vi "Main.vi"() -> ()   [LabVIEW 2018]
uses:
  Data Def/Main State.ctl
  Data Def/Tips.ctl
  Data Def/Frequency Setting.ctl
  Data Def/Subpanel State.ctl
  Data Def/Channel Count.ctl
  Data Def/Signal Type Setting.ctl
  Function/Data Def/Voice Control Reference.ctl
  Data Def/Loop Control Command.ctl
  Data Def/Main Loop Command.ctl
  Data Def/Parameter.ctl
  <vilib>/Utility/miscctls.llb/LVPositionTypeDef.ctl
panel:
  in  "Setting Parameter":bool
  in  "Get Data":bool
  in  "Menue":bool
  in  "Score":dbl
  out "Voice Chatt":dbl(graph)
  out "Voice":string
  out "Voice State":bool
  in  "Stop":bool
  in  "Tab Control 2":enum32{"Page 1"}(tab)
  out "Tips":T1
  in  "Help":bool
  out "Main Tab":T2
  in  "Save":bool
  in  "Previous Page":bool
  out "SubTab":T3
  in  "Signal Type":bool
  in  "Channel":bool
  in  "Frequency":bool
  in  "Frequency Setting":T4 caption="頻率"
  in  "Channel Count":T5 caption="通道數"
  in  "Signal Type Setting":T6 caption="波形"
  in  "Switch":bool
  out "Spectrum":cluster{"f0":dbl, "df":dbl, "magnitude":dbl[]}[](graph)
  out "Wave":waveform(dbl)[](graph)
  # "微軟語音辨識軟體動後，請對軟體說出每個\n按鈕的名稱或由左方按鍵手動操作。"
  # "目錄"
  # "請確定微軟語音辨識軟體有正確開啟並運作。"
  # "請選擇以下功能"
  # "設定參數"
  # "擷取數據"
  # "擷取數據"
  # "幫助"
  # "停止"
  # "開/關"
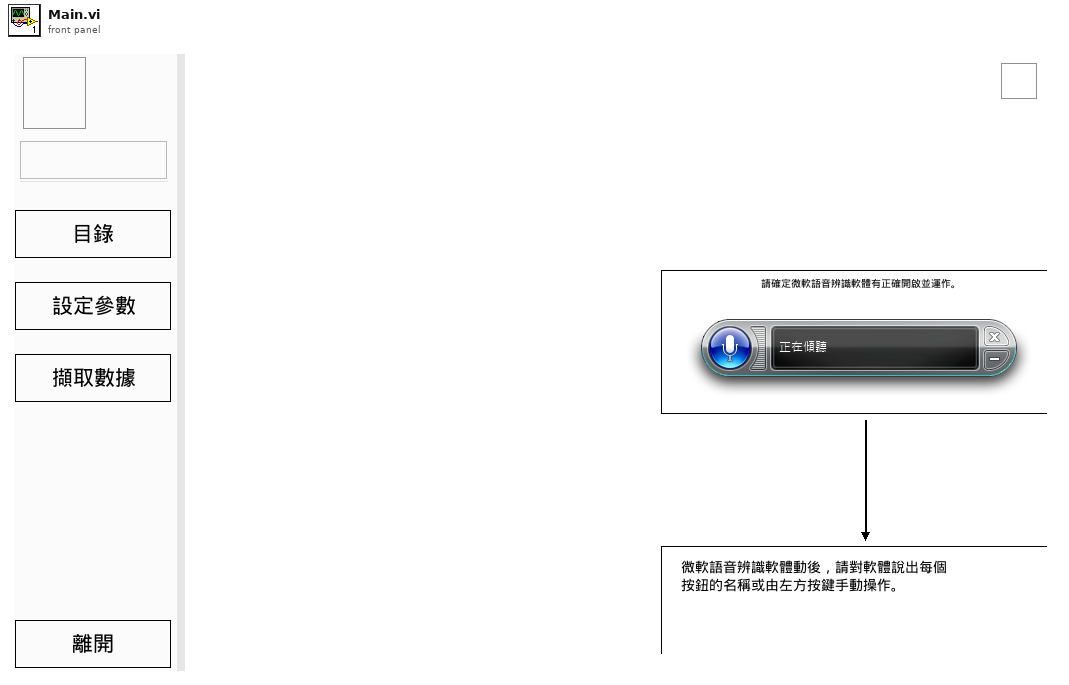
[diagram p1: front panel]
types:
  T1 = typedef "Tips.ctl" = string
  T2 = typedef "Main State.ctl" = enum32{"Initialize", "Start", "Set Parameter", "Get Data"}
  T3 = typedef "Subpanel State.ctl" = enum32{"Main", "Frequency", "Count of Channel", "Signal Type"}
  T4 = typedef "Frequency Setting.ctl" = enum32{"10 Hz", "50 Hz", "100 Hz"}
  T5 = typedef "Channel Count.ctl" = enum32{"1", "2", "3", "4"}
  T6 = typedef "Signal Type Setting.ctl" = enum32{"Sine", "Sqaure", "Triangle"}
  T7 = typedef "Main Loop Command.ctl" = enum16{"Initialize", "Menue", "Setting Parameter", "Get Data", "Help", "Frequency", "Channel", "Signal Type", "Previous Page", "Save", "Exit"}
  T8 = typedef "Loop Control Command.ctl" = enum16{"Initialize", "Enqueue", "Insert", "Flush", "Release"}
  T9 = typedef "Voice Control Reference.ctl" = cluster{"String in":refnum<vi>, "Score in":refnum<vi>}
  T10 = typedef "Callback Event Reference.ctl" = cluster{"new reference":refnum<k24>, "Event Callback":refnum<k27>}
  T11 = enum32{"Main", "Frequency", "Count of Channel", "Signal Type"}
  T12 = typedef "Parameter.ctl" = cluster{"Channel Count":T5, "Frequency Setting":T4, "Signal Type Setting":T6}
  T13 = enum16{"Save File", "Read File", "Put Frequency", "Put Signal Type", "Put Channel", "Put All", "Get All"}
  T14 = typedef "LVPositionTypeDef.ctl" = cluster{"Left":i32, "Top":i32}
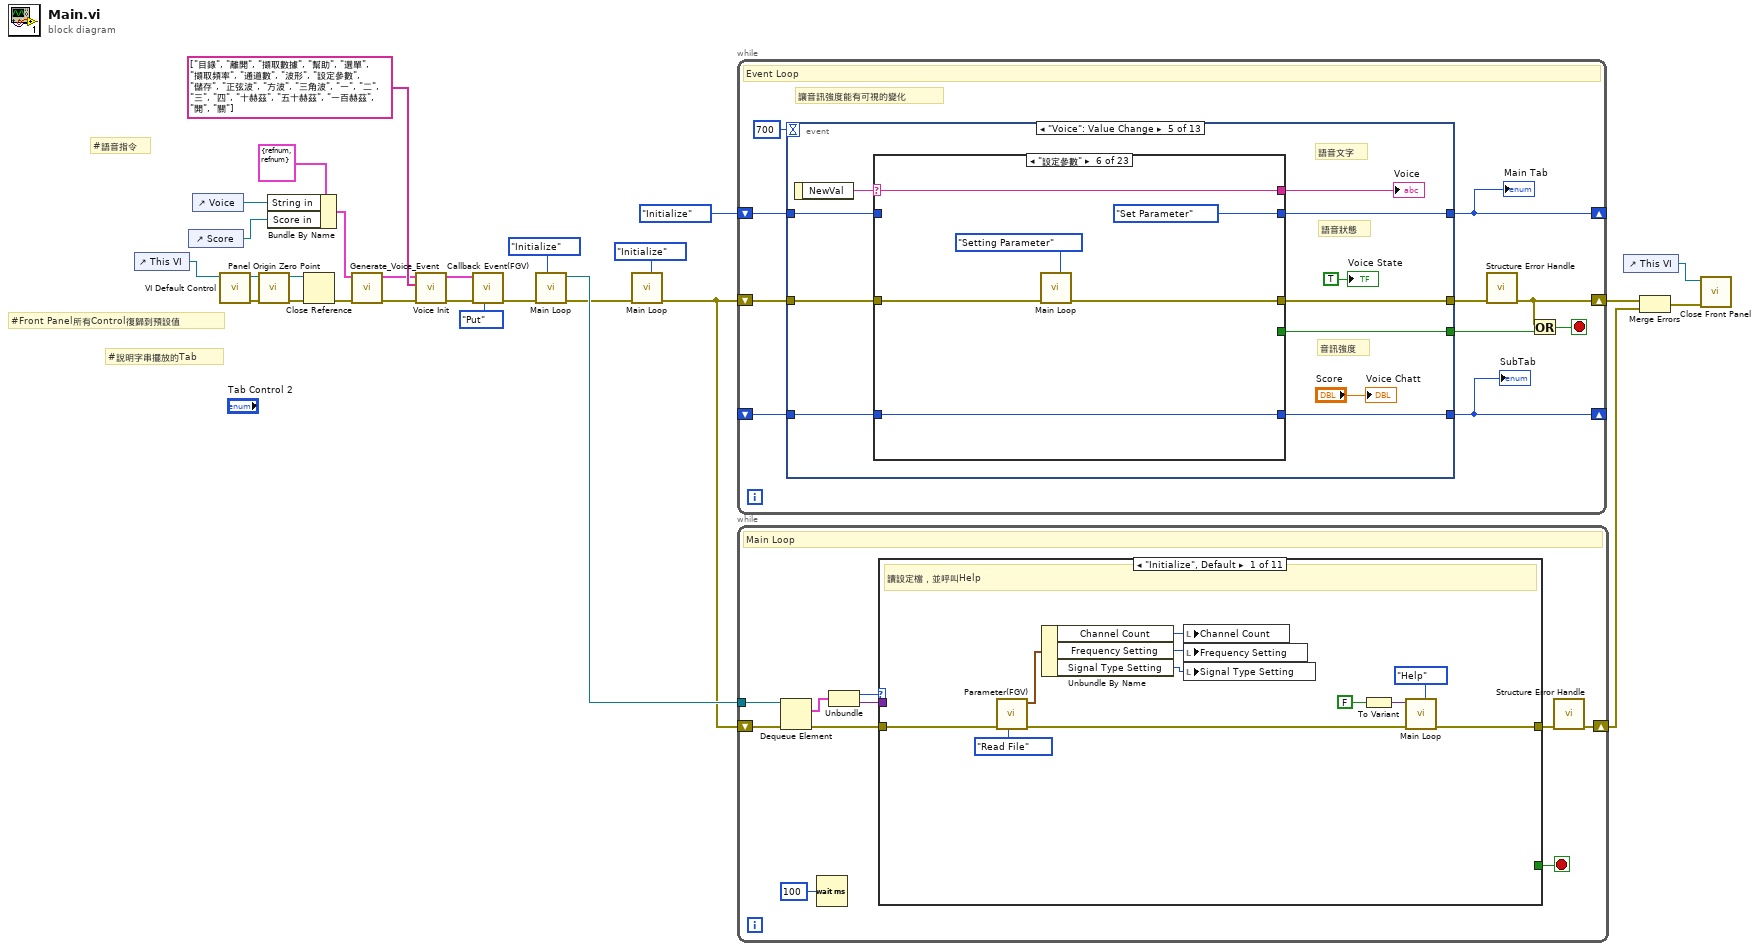
[diagram p0: block diagram]
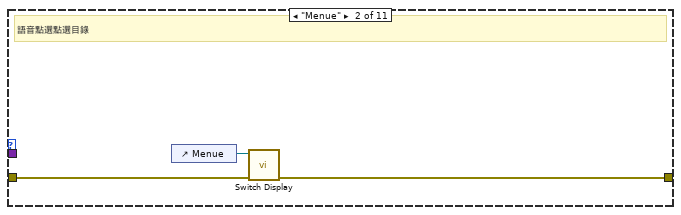
[diagram p2: hidden frame]
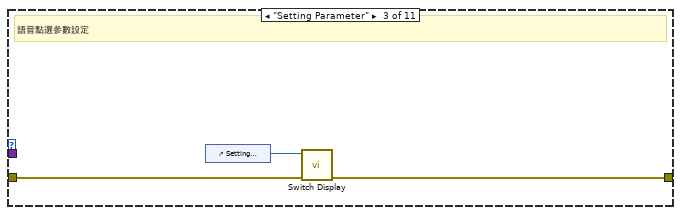
[diagram p3: hidden frame]
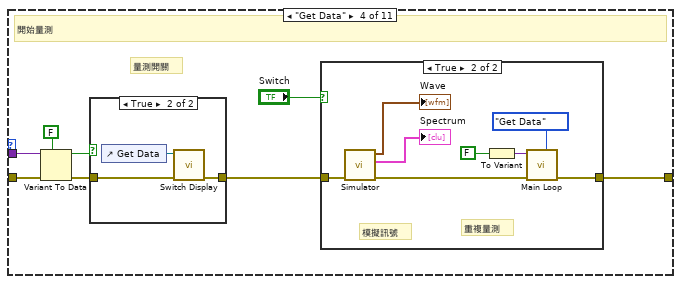
[diagram p4: hidden frame]
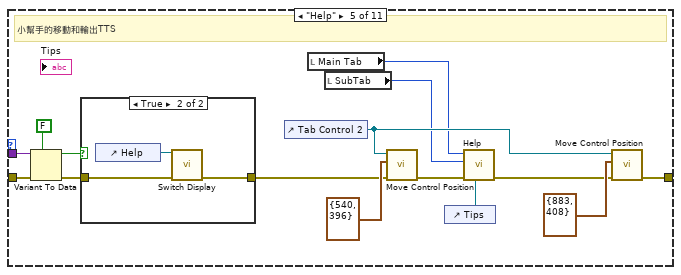
[diagram p7: hidden frame]
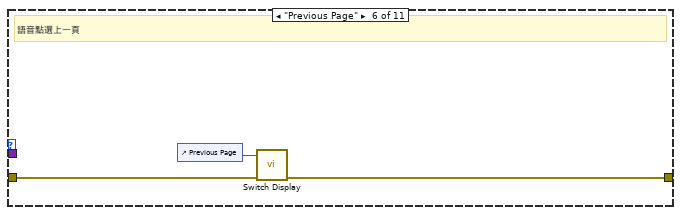
[diagram p9: hidden frame]
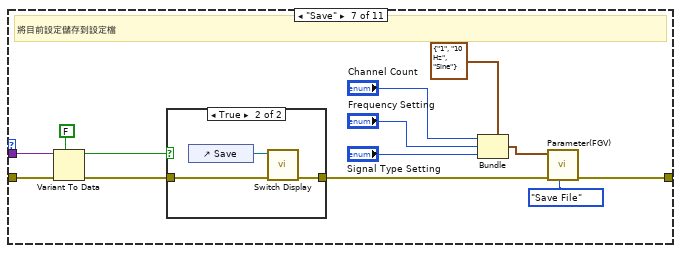
[diagram p10: hidden frame]
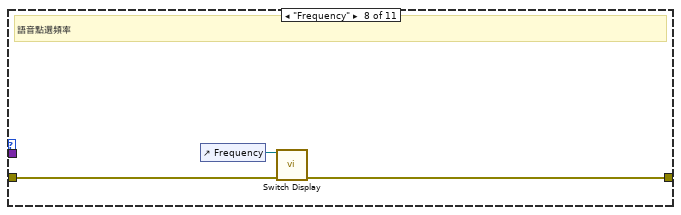
[diagram p12: hidden frame]
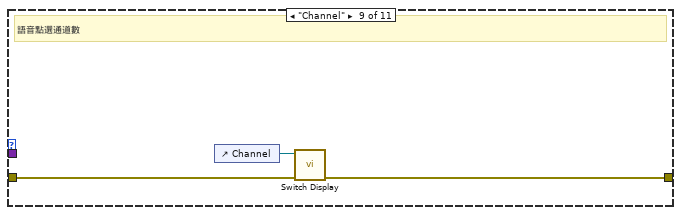
[diagram p13: hidden frame]
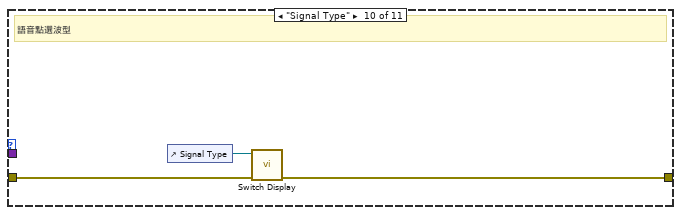
[diagram p14: hidden frame]
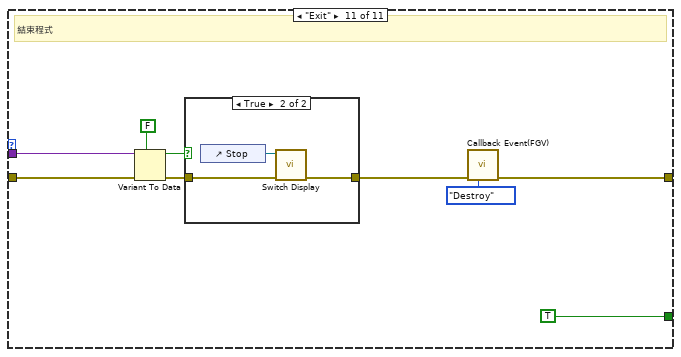
[diagram p15: hidden frame]
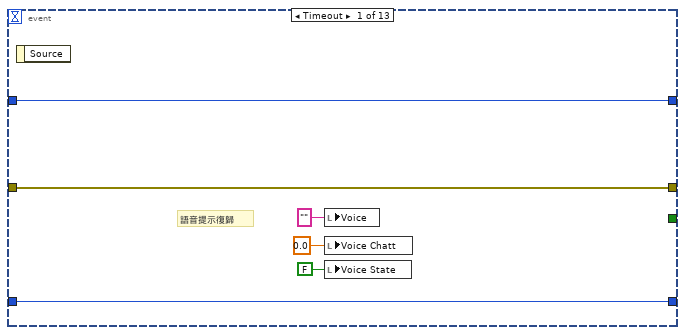
[diagram p17: hidden frame]
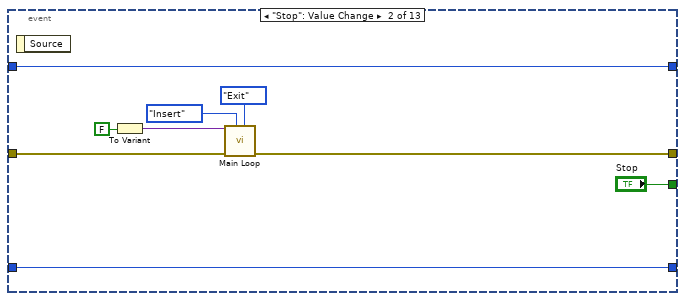
[diagram p18: hidden frame]
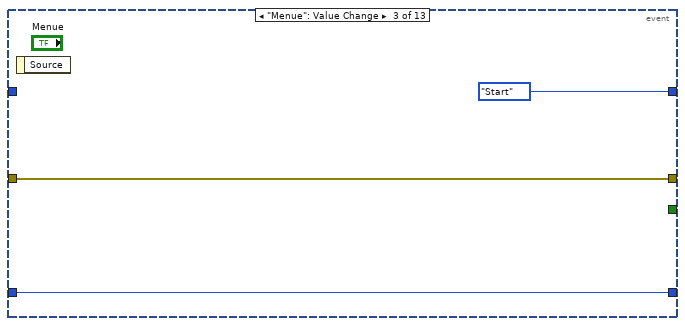
[diagram p19: hidden frame]
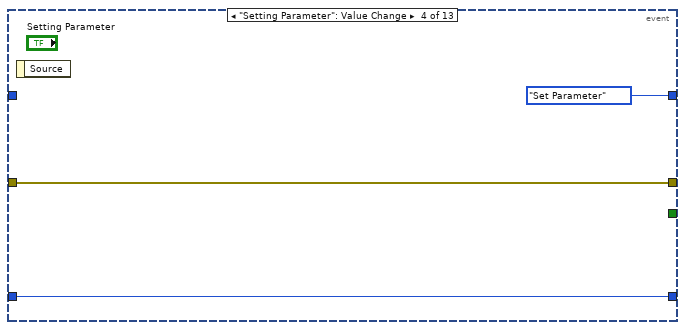
[diagram p20: hidden frame]
diagram:
  # "#Front Panel所有Control復歸到預設值"
  # "#語音指令"
  # "#說明字串擺放的Tab"
  n1 = control-ref of="This VI"() -> (w10:refnum<vi>)
  n2 = control-ref of="Score"() -> (w25:refnum<vi>)
  n3 = control-ref of="Voice"() -> (w26:refnum<vi>)
  n4 = call "VI Default Control.vi"("VI Reference in"=w10) -> ("error out"=w9:errorcluster, "VI Reference out"=w8:refnum<vi>)  [unwired: 9 in]
  n5 = call "Panel Origin Zero Point.vi"("error in"=w9, "VI Reference In"=w8) -> ("error out"=w7:errorcluster, "VI Reference Out"=w6:refnum<vi>)  [unwired: 8 in]
  n6 = Bundle By Name(cluster=T9 {"String in"=refnum, "Score in"=refnum} ("Voice Control Reference In"), "String in"=w26, "Score in"=w25) -> (w24:T9)
  n7 = Close Reference(reference=w6, error in (no error)=w7) -> (error out=w5:errorcluster)
  n8 = call "Generate_Voice_Event.vi"("Error In"=w5, "Voice Control Reference In"=w24) -> ("Error Out"=w23:errorcluster, "Voice Control Reference Out"=w21:T9)  [unwired: 8 in]
  n9 = call "Voice Init.vi"("Error In"=w23, "CMD List"=string[] ["目錄", "離開", "擷取數據", "幫助", "選單", "擷取頻率", "通道數", "波形", "設定參數", "儲存", "正弦波", "方波", "三角波", "一", "二", "三", "四", "十赫茲", "五十赫茲", "一百赫茲", "開", "關"] ("String[] phrases"), "Main Control Reference"=w21) -> ("Error Out"=w20:errorcluster, "Callback Event Reference"=w19:T10)  [unwired: 7 in]
  n10 = call "Callback Event(FGV).vi"("Method"=enum16{"Destroy", "Put", "Get"}."Put", "error in"=w20, "Callback Event Reference In"=w19) -> ("error out"=w11:errorcluster)  [unwired: 7 in, 1 out]
  n11 = call "Main Loop.vi"("Loop cotrol command"=Loop_Control_Command."Initialize", "error in"=w11) -> ("error out"=w14:errorcluster, "Main Queue"=w16:refnum<queue>)  [unwired: 8 in]
  n12 = call "Main Loop.vi"("Main Loop Command"=Main_Loop_Command."Initialize", "error in"=w14) -> ("error out"=w13:errorcluster)  [unwired: 8 in, 1 out]
  n13 = while {
    shift-right: [w28] -> w4
    shift-left: w13 -> [w36]
    shift-right: [w32] -> _
    shift-left: Main_State."Initialize" ("Tab Control") -> [w33]
    shift-right: [w31] -> _
    shift-left: _ -> [w30]
    stop <- w34 stop-if-true
    # "讓音訊強度能有可視的變化"
    # "Event Loop"
    n14 = event shown="[4] \"Voice\": Value Change" {
      selector: _ -> [_ _ _ _ _ _ _ _ _ _ _ _ _]
      dyn-events: _ -> [_ _ _ _ _ _ _ _ _ _ _ _ _]
      timeout: 700 -> [_ _ _ _ _ _ _ _ _ _ _ _ _]
      tunnel: w36 -> [w43 w51 w53 w56 w66 w254 w264 w274 w276 w279 w283 w288 w298]
      tunnel: [w43 w50 w53 w56 w67 w253 w263 w274 w276 w279 w283 w287 w296] -> w29
      tunnel: [_ "Stop" _ _ w65 _ _ _ _ _ _ _ _] -> w35
      tunnel: w33 -> [w40 w48 _ _ w62 _ w265 w273 w277 w280 w282 w286 w295]
      tunnel: [w40 w48 Main_State."Start" ("Tab Control") Main_State."Set Parameter" ("Tab Control") w61 Main_State."Get Data" ("Tab Control") w265 w273 w277 w280 w282 w286 w295] -> w32
      tunnel: [w38 w44 w54 w57 w60 w251 w262 Subpanel_State."Main" ("SubTab") Subpanel_State."Frequency" ("SubTab") Subpanel_State."Count of Channel" ("SubTab") Subpanel_State."Signal Type" ("SubTab") Subpanel_State."Main" ("SubTab") w299] -> w31
      tunnel: w30 -> [w38 w44 w54 w57 w59 w251 w262 _ _ _ _ _ w299]
      event Timeout {
        # "語音提示復歸"
        n15 = event-data() -> ()  [unwired: 1 in, 1 out]
        n16 = local write "Voice"("" ("Voice")) -> ()
        n17 = local write "Voice Chatt"(0.0 ("Voice Intensity")) -> ()
        n18 = local write "Voice State"(FALSE ("Voice State")) -> ()
      }
      event "Stop": Value Change {
        n19 = event-data() -> ()  [unwired: 1 in, 1 out]
        n20 = To Variant(anything=FALSE) -> (Variant=w45:variant)
        n21 = call "Main Loop.vi"("Main Loop Command"=Main_Loop_Command."Exit", "Loop cotrol command"=Loop_Control_Command."Insert", "error in"=w51, "Data"=w45) -> ("error out"=w50:errorcluster)  [unwired: 6 in, 1 out]
      }
      event "Menue": Value Change {
        n22 = event-data() -> ()  [unwired: 1 in, 1 out]
      }
      event "Setting Parameter": Value Change {
        n23 = event-data() -> ()  [unwired: 1 in, 1 out]
      }
      event "Voice": Value Change {
        # "音訊強度"
        # "語音狀態"
        # "語音文字"
        n24 = event-data() -> ("NewVal"=w69:string)  [unwired: 1 in]
        n25 = case shown="\"設定參數\"" w69 {
          selector: w69 -> [_ w81 w91 w99 w107 w113 w119 w121 w128 w133 w138 w153 w161 w170 w179 w188 w197 w206 w215 w224 w233 w236 w247]
          tunnel: ["再說一次 " w81 w91 w99 w107 w113 w119 w121 w128 w133 w138 w153 w161 w170 w179 w188 w197 w206 w215 w224 w233 w236 w247] -> w68
          tunnel: [w73 w78 w89 w98 w104 w110 w115 w124 w129 w135 w142 w149 w156 w164 w175 w182 w191 w200 w209 w218 w227 w238 w245] -> w67
          tunnel: w66 -> [w73 w79 w85 w95 w105 w112 w116 w125 w130 w136 w143 w150 w157 w165 w176 w183 w192 w201 w210 w219 w228 w239 w245]
          tunnel: [_ _ TRUE _ _ _ _ _ _ _ _ _ _ _ _ _ _ _ _ _ _ _ _] -> w65
          tunnel: w62 -> [w72 _ w87 _ w106 _ w118 w122 w127 w134 w144 w152 w163 w172 w181 w190 w199 w208 w217 w226 w235 w244 w249]
          tunnel: [w72 Main_State."Start" ("Tab Control") w87 Main_State."Get Data" ("Tab Control") w106 Main_State."Set Parameter" ("Tab Control") w118 w122 w127 w134 w144 w152 w163 w172 w181 w190 w199 w208 w217 w226 w235 w244 w249] -> w61
          tunnel: [w70 w74 w82 w92 w100 w108 T11."Main" ("SubTab") T11."Frequency" ("SubTab") T11."Count of Channel" ("SubTab") T11."Signal Type" ("SubTab") w145 w154 w162 w171 w180 w189 w198 w207 w216 w225 w234 w243 w248] -> w60
          tunnel: w59 -> [w70 w74 w82 w92 w100 w108 _ _ _ _ w145 w154 w162 w171 w180 w189 w198 w207 w216 w225 w234 w243 w248]
          frame Default {
          }
          frame "目錄" {
            n26 = To Variant(anything=TRUE) -> (Variant=w77:variant)
            n27 = call "Main Loop.vi"("Main Loop Command"=Main_Loop_Command."Menue", "error in"=w79, "Data"=w77) -> ("error out"=w78:errorcluster)  [unwired: 7 in, 1 out]
          }
          frame "離開" {
            n28 = To Variant(anything=TRUE) -> (Variant=w84:variant)
            n29 = call "Main Loop.vi"("Main Loop Command"=Main_Loop_Command."Exit", "Loop cotrol command"=Loop_Control_Command."Insert", "error in"=w85, "Data"=w84) -> ("error out"=w89:errorcluster)  [unwired: 6 in, 1 out]
          }
          frame "擷取數據" {
            n30 = To Variant(anything=TRUE) -> (Variant=w94:variant)
            n31 = call "Main Loop.vi"("Main Loop Command"=Main_Loop_Command."Get Data", "error in"=w95, "Data"=w94) -> ("error out"=w98:errorcluster)  [unwired: 7 in, 1 out]
          }
          frame "幫助" {
            n32 = To Variant(anything=TRUE) -> (Variant=w101:variant)
            n33 = call "Main Loop.vi"("Main Loop Command"=Main_Loop_Command."Help", "error in"=w105, "Data"=w101) -> ("error out"=w104:errorcluster)  [unwired: 7 in, 1 out]
          }
          frame "設定參數" {
            n34 = call "Main Loop.vi"("Main Loop Command"=Main_Loop_Command."Setting Parameter", "error in"=w112) -> ("error out"=w110:errorcluster)  [unwired: 8 in, 1 out]
          }
          frame "選單" {
            n35 = call "Main Loop.vi"("Main Loop Command"=Main_Loop_Command."Previous Page", "error in"=w116) -> ("error out"=w115:errorcluster)  [unwired: 8 in, 1 out]
          }
          frame "擷取頻率" {
            n36 = call "Main Loop.vi"("Main Loop Command"=Main_Loop_Command."Frequency", "error in"=w125) -> ("error out"=w124:errorcluster)  [unwired: 8 in, 1 out]
          }
          frame "通道數" {
            n37 = call "Main Loop.vi"("Main Loop Command"=Main_Loop_Command."Channel", "error in"=w130) -> ("error out"=w129:errorcluster)  [unwired: 8 in, 1 out]
          }
          frame "波形" {
            n38 = call "Main Loop.vi"("Main Loop Command"=Main_Loop_Command."Channel", "error in"=w136) -> ("error out"=w135:errorcluster)  [unwired: 8 in, 1 out]
          }
          frame "儲存" {
            n39 = To Variant(anything=TRUE) -> (Variant=w139:variant)
            n40 = call "Main Loop.vi"("Main Loop Command"=Main_Loop_Command."Save", "error in"=w143, "Data"=w139) -> ("error out"=w142:errorcluster)  [unwired: 7 in, 1 out]
          }
          frame "正弦波" {
            w146 = Signal_Type_Setting."Sine" ("Signal Type Setting")
            n41 = Bundle By Name(cluster=T12 {"Channel Count"=enum."1", "Frequency Setting"=enum."10 Hz", "Signal Type Setting"=enum."Sine"} ("Parameter In"), "Signal Type Setting"=w146) -> (w147:T12)
            n42 = local write "Signal Type Setting"(w146) -> ()
            n43 = call "Parameter(FGV).vi"("Parameter Method"=T13."Put Signal Type", "error in"=w150, "Parameter In"=w147) -> ("error out"=w149:errorcluster)  [unwired: 7 in, 1 out]
          }
          frame "三角波" {
            w155 = Signal_Type_Setting."Triangle" ("Signal Type Setting")
            n44 = Bundle By Name(cluster=T12 {"Channel Count"=enum."1", "Frequency Setting"=enum."10 Hz", "Signal Type Setting"=enum."Sine"} ("Parameter In"), "Signal Type Setting"=w155) -> (w158:T12)
            n45 = local write "Signal Type Setting"(w155) -> ()
            n46 = call "Parameter(FGV).vi"("Parameter Method"=T13."Put Signal Type", "error in"=w157, "Parameter In"=w158) -> ("error out"=w156:errorcluster)  [unwired: 7 in, 1 out]
          }
          frame "方波" {
            w166 = Signal_Type_Setting."Sqaure" ("Signal Type Setting")
            n47 = Bundle By Name(cluster=T12 {"Channel Count"=enum."1", "Frequency Setting"=enum."10 Hz", "Signal Type Setting"=enum."Sine"} ("Parameter In"), "Signal Type Setting"=w166) -> (w167:T12)
            n48 = local write "Signal Type Setting"(w166) -> ()
            n49 = call "Parameter(FGV).vi"("Parameter Method"=T13."Put Signal Type", "error in"=w165, "Parameter In"=w167) -> ("error out"=w164:errorcluster)  [unwired: 7 in, 1 out]
          }
          frame "十赫茲" {
            w173 = Frequency_Setting."10 Hz" ("Frequency Setting")
            n50 = Bundle By Name(cluster=T12 {"Channel Count"=enum."1", "Frequency Setting"=enum."10 Hz", "Signal Type Setting"=enum."Sine"} ("Parameter In"), "Frequency Setting"=w173) -> (w177:T12)
            n51 = local write "Frequency Setting"(w173) -> ()
            n52 = call "Parameter(FGV).vi"("Parameter Method"=T13."Put Frequency", "error in"=w176, "Parameter In"=w177) -> ("error out"=w175:errorcluster)  [unwired: 7 in, 1 out]
          }
          frame "五十赫茲" {
            w184 = Frequency_Setting."50 Hz" ("Frequency Setting")
            n53 = Bundle By Name(cluster=T12 {"Channel Count"=enum."1", "Frequency Setting"=enum."10 Hz", "Signal Type Setting"=enum."Sine"} ("Parameter In"), "Frequency Setting"=w184) -> (w186:T12)
            n54 = local write "Frequency Setting"(w184) -> ()
            n55 = call "Parameter(FGV).vi"("Parameter Method"=T13."Put Frequency", "error in"=w183, "Parameter In"=w186) -> ("error out"=w182:errorcluster)  [unwired: 7 in, 1 out]
          }
          frame "一百赫茲" {
            w193 = Frequency_Setting."100 Hz" ("Frequency Setting")
            n56 = Bundle By Name(cluster=T12 {"Channel Count"=enum."1", "Frequency Setting"=enum."10 Hz", "Signal Type Setting"=enum."Sine"} ("Parameter In"), "Frequency Setting"=w193) -> (w195:T12)
            n57 = local write "Frequency Setting"(w193) -> ()
            n58 = call "Parameter(FGV).vi"("Parameter Method"=T13."Put Frequency", "error in"=w192, "Parameter In"=w195) -> ("error out"=w191:errorcluster)  [unwired: 7 in, 1 out]
          }
          frame "一" {
            w205 = Channel_Count."1" ("Channel Count")
            n59 = Bundle By Name(cluster=T12 {"Channel Count"=enum."1", "Frequency Setting"=enum."10 Hz", "Signal Type Setting"=enum."Sine"} ("Parameter In"), "Channel Count"=w205) -> (w203:T12)
            n60 = local write "Channel Count"(w205) -> ()
            n61 = call "Parameter(FGV).vi"("Parameter Method"=T13."Put Channel", "error in"=w201, "Parameter In"=w203) -> ("error out"=w200:errorcluster)  [unwired: 7 in, 1 out]
          }
          frame "二" {
            w214 = Channel_Count."2" ("Channel Count")
            n62 = Bundle By Name(cluster=T12 {"Channel Count"=enum."1", "Frequency Setting"=enum."10 Hz", "Signal Type Setting"=enum."Sine"} ("Parameter In"), "Channel Count"=w214) -> (w212:T12)
            n63 = local write "Channel Count"(w214) -> ()
            n64 = call "Parameter(FGV).vi"("Parameter Method"=T13."Put Channel", "error in"=w210, "Parameter In"=w212) -> ("error out"=w209:errorcluster)  [unwired: 7 in, 1 out]
          }
          frame "三" {
            w223 = Channel_Count."3" ("Channel Count")
            n65 = Bundle By Name(cluster=T12 {"Channel Count"=enum."1", "Frequency Setting"=enum."10 Hz", "Signal Type Setting"=enum."Sine"} ("Parameter In"), "Channel Count"=w223) -> (w221:T12)
            n66 = local write "Channel Count"(w223) -> ()
            n67 = call "Parameter(FGV).vi"("Parameter Method"=T13."Put Channel", "error in"=w219, "Parameter In"=w221) -> ("error out"=w218:errorcluster)  [unwired: 7 in, 1 out]
          }
          frame "四" {
            w232 = Channel_Count."4" ("Channel Count")
            n68 = Bundle By Name(cluster=T12 {"Channel Count"=enum."1", "Frequency Setting"=enum."10 Hz", "Signal Type Setting"=enum."Sine"} ("Parameter In"), "Channel Count"=w232) -> (w230:T12)
            n69 = local write "Channel Count"(w232) -> ()
            n70 = call "Parameter(FGV).vi"("Parameter Method"=T13."Put Channel", "error in"=w228, "Parameter In"=w230) -> ("error out"=w227:errorcluster)  [unwired: 7 in, 1 out]
          }
          frame "開" {
            n71 = To Variant(anything=FALSE) -> (Variant=w241:variant)
            n72 = call "Main Loop.vi"("Main Loop Command"=Main_Loop_Command."Get Data", "error in"=w239, "Data"=w241) -> ("error out"=w238:errorcluster)  [unwired: 7 in, 1 out]
            n73 = local write "Switch"(TRUE ("Switch")) -> ()
          }
          frame "關" {
            n74 = local write "Switch"(FALSE ("Switch")) -> ()
          }
        }
        "Voice" <- w68
        "Voice State" <- TRUE ("Voice State")
        "Voice Chatt" <- "Score"
      }
      event "Get Data": Value Change {
        n75 = event-data() -> ()  [unwired: 1 in, 1 out]
        n76 = case shown="True" "Get Data" {
          tunnel: w254 -> [w255 w260]
          tunnel: [w255 w259] -> w253
          frame False {
          }
          frame True {
            n77 = To Variant(anything=FALSE) -> (Variant=w257:variant)
            n78 = call "Main Loop.vi"("Main Loop Command"=Main_Loop_Command."Get Data", "error in"=w260, "Data"=w257) -> ("error out"=w259:errorcluster)  [unwired: 7 in, 1 out]
          }
        }
      }
      event "Help": Value Change {
        n79 = event-data() -> ()  [unwired: 1 in, 1 out]
        n80 = case shown="True" "Help" {
          tunnel: w264 -> [w266 w271]
          tunnel: [w266 w270] -> w263
          frame False {
          }
          frame True {
            n81 = To Variant(anything=FALSE) -> (Variant=w267:variant)
            n82 = call "Main Loop.vi"("Main Loop Command"=Main_Loop_Command."Help", "error in"=w271, "Data"=w267) -> ("error out"=w270:errorcluster)  [unwired: 7 in, 1 out]
          }
        }
      }
      event "Previous Page": Value Change {
        n83 = event-data() -> ()  [unwired: 1 in, 1 out]
      }
      event "Frequency": Value Change {
        n84 = event-data() -> ()  [unwired: 1 in, 1 out]
      }
      event "Channel": Value Change {
        n85 = event-data() -> ()  [unwired: 1 in, 1 out]
      }
      event "Signal Type": Value Change {
        n86 = event-data() -> ()  [unwired: 1 in, 1 out]
      }
      event "Save": Value Change {
        n87 = event-data() -> ()  [unwired: 1 in, 1 out]
        n88 = case shown="True" "Save" {
          tunnel: w288 -> [w289 w291]
          tunnel: [w289 w290] -> w287
          frame False {
          }
          frame True {
            n89 = To Variant(anything=FALSE) -> (Variant=w292:variant)
            n90 = call "Main Loop.vi"("Main Loop Command"=Main_Loop_Command."Save", "error in"=w291, "Data"=w292) -> ("error out"=w290:errorcluster)  [unwired: 7 in, 1 out]
          }
        }
      }
      event "Switch": Value Change {
        n91 = event-data() -> ("NewVal"=w297:bool)  [unwired: 1 in]
        n92 = case shown="True" w297 {
          tunnel: w298 -> [w300 w302]
          tunnel: [w300 w301] -> w296
          frame False {
          }
          frame True {
            n93 = To Variant(anything=FALSE) -> (Variant=w304:variant)
            n94 = call "Main Loop.vi"("Main Loop Command"=Main_Loop_Command."Get Data", "error in"=w302, "Data"=w304) -> ("error out"=w301:errorcluster)  [unwired: 7 in, 1 out]
          }
        }
      }
    }
    "Main Tab" <- w32
    "SubTab" <- w31
    n95 = call "Structure Error Handle.vi"("error in"=w29) -> ("error out"=w28:errorcluster)  [unwired: 10 in]
    n96 = Or(x=w28, y=w35) -> (x .or. y?=w34:bool)
  }
  n97 = while {
    tunnel: w16 -> [w314]
    shift-right: [w306] -> w3
    shift-left: w13 -> [w315]
    stop <- w310 stop-if-true
    # "Main Loop"
    n98 = Dequeue Element(queue=w314, error in (no error)=w315) -> (element=w313:cluster{"Main Loop Command":T7, "Data":variant}, error out=w311:errorcluster)  [unwired: 1 in, 2 out]
    n99 = Wait (ms)(milliseconds to wait=u32 100) -> ()  [unwired: 1 out]
    n100 = Unbundle(w313) -> ("Main Loop Command"=w312:T7, "Data"=w309:variant)
    n101 = case shown="\"Initialize\", Default" w312 {
      tunnel: w311 -> [w321 w327 w332 w339 w361 w373 w384 w393 w397 w401 w408]
      tunnel: [w318 w329 w331 w340 w365 w375 w386 w395 w398 w400 w402] -> w307
      tunnel: [_ _ _ _ _ _ _ _ _ _ TRUE] -> w310
      tunnel: w309 -> [_ _ _ w338 w359 _ w383 _ _ _ w407]
      frame "Initialize", Default {
        # "讀設定檔，並呼叫Help"
        n102 = call "Parameter(FGV).vi"("Parameter Method"=T13."Read File", "error in"=w321) -> ("error out"=w320:errorcluster, "Parameter Out"=w324:T12)  [unwired: 8 in]
        n103 = Unbundle By Name(w324) -> ("Channel Count"=w325:T5, "Frequency Setting"=w326:T4, "Signal Type Setting"=w322:T6)
        n104 = local write "Channel Count"(w325) -> ()
        n105 = local write "Frequency Setting"(w326) -> ()
        n106 = local write "Signal Type Setting"(w322) -> ()
        n107 = To Variant(anything=FALSE) -> (Variant=w316:variant)
        n108 = call "Main Loop.vi"("Main Loop Command"=Main_Loop_Command."Help", "error in"=w320, "Data"=w316) -> ("error out"=w318:errorcluster)  [unwired: 7 in, 1 out]
      }
      frame "Menue" {
        # "語音點選點選目錄"
        n109 = control-ref of="Menue"() -> (w328:refnum<vi>)
        n110 = call "Switch Display.vi"("error in"=w327, "Boolean"=w328) -> ("error out"=w329:errorcluster)  [unwired: 9 in]
      }
      frame "Setting Parameter" {
        # "語音點選參數設定"
        n111 = control-ref of="Setting Parameter"() -> (w330:refnum<vi>)
        n112 = call "Switch Display.vi"("error in"=w332, "Boolean"=w330) -> ("error out"=w331:errorcluster)  [unwired: 9 in]
      }
      frame "Get Data" {
        # "量測開關"
        # "開始量測"
        n113 = Variant To Data(error in=w339, type=FALSE, Variant=w338) -> (data=w335:bool, error out=w337:errorcluster)
        n114 = case shown="True" w335 {
          tunnel: w337 -> [w350 w353]
          tunnel: [w350 w352] -> w334
          frame False {
          }
          frame True {
            n115 = control-ref of="Get Data"() -> (w351:refnum<vi>)
            n116 = call "Switch Display.vi"("error in"=w353, "Boolean"=w351) -> ("error out"=w352:errorcluster)  [unwired: 9 in]
          }
        }
        n117 = case shown="True" "Switch" {
          tunnel: [w341 w348] -> w340
          tunnel: w334 -> [w341 w345]
          frame False {
          }
          frame True {
            # "重複量測"
            # "模擬訊號"
            n118 = call "Simulator.vi"("error in"=w345) -> ("error out"=w342:errorcluster, "FFT"=→"Spectrum":cluster{"f0":dbl, "df":dbl, "magnitude":dbl[]}[], "Wave"=→"Wave":waveform(dbl)[])  [unwired: 8 in]
            n119 = To Variant(anything=FALSE) -> (Variant=w347:variant)
            n120 = call "Main Loop.vi"("Main Loop Command"=Main_Loop_Command."Get Data", "error in"=w342, "Data"=w347) -> ("error out"=w348:errorcluster)  [unwired: 7 in, 1 out]
          }
        }
      }
      frame "Help" {
        # "小幫手的移動和輸出TTS"
        n121 = Variant To Data(error in=w361, type=FALSE, Variant=w359) -> (data=w362:bool, error out=w364:errorcluster)
        n122 = case shown="True" w362 {
          tunnel: w364 -> [w369 w372]
          tunnel: [w369 w371] -> w360
          frame False {
          }
          frame True {
            n123 = control-ref of="Help"() -> (w370:refnum<vi>)
            n124 = call "Switch Display.vi"("error in"=w372, "Boolean"=w370) -> ("error out"=w371:errorcluster)  [unwired: 9 in]
          }
        }
        n125 = control-ref of="Tab Control 2"() -> (w366:refnum<vi>)
        n126 = local read "Main Tab"() -> (w355:T2)
        n127 = local read "SubTab"() -> (w356:T3)
        n128 = call "Move Control Position.vi"("error in (no error)"=w360, "Desired Position"=T14 {"Left"=540, "Top"=396} ("Position"), "Obj Ref"=w366) -> ("error out"=w358:errorcluster)  [unwired: 6 in, 2 out]
        n129 = control-ref of="Tips"() -> (w354:refnum<vi>)
        n130 = call "Help.vi"("reference"=w354, "error in"=w358, "SubTab"=w356, "Tab Control"=w355) -> ("error out"=w357:errorcluster)  [unwired: 7 in]
        n131 = call "Move Control Position.vi"("error in (no error)"=w357, "Desired Position"=T14 {"Left"=883, "Top"=408} ("Position"), "Obj Ref"=w366) -> ("error out"=w365:errorcluster)  [unwired: 6 in, 2 out]
      }
      frame "Previous Page" {
        # "語音點選上一頁"
        n132 = control-ref of="Previous Page"() -> (w374:refnum<vi>)
        n133 = call "Switch Display.vi"("error in"=w373, "Boolean"=w374) -> ("error out"=w375:errorcluster)  [unwired: 9 in]
      }
      frame "Save" {
        # "將目前設定儲存到設定檔"
        n134 = Variant To Data(error in=w384, type=FALSE, Variant=w383) -> (data=w382:bool, error out=w381:errorcluster)
        n135 = case shown="True" w382 {
          tunnel: [w389 w391] -> w387
          tunnel: w381 -> [w389 w390]
          frame False {
          }
          frame True {
            n136 = control-ref of="Save"() -> (w392:refnum<vi>)
            n137 = call "Switch Display.vi"("error in"=w390, "Boolean"=w392) -> ("error out"=w391:errorcluster)  [unwired: 9 in]
          }
        }
        n138 = Bundle(cluster=T12 {"Channel Count"=enum."1", "Frequency Setting"=enum."10 Hz", "Signal Type Setting"=enum."Sine"} ("Parameter In"), "Channel Count"="Channel Count", "Frequency Setting"="Frequency Setting", "Signal Type Setting"="Signal Type Setting") -> (w376:T12)
        n139 = call "Parameter(FGV).vi"("Parameter Method"=T13."Save File", "error in"=w387, "Parameter In"=w376) -> ("error out"=w386:errorcluster)  [unwired: 7 in, 1 out]
      }
      frame "Frequency" {
        # "語音點選頻率"
        n140 = control-ref of="Frequency"() -> (w394:refnum<vi>)
        n141 = call "Switch Display.vi"("error in"=w393, "Boolean"=w394) -> ("error out"=w395:errorcluster)  [unwired: 9 in]
      }
      frame "Channel" {
        # "語音點選通道數"
        n142 = control-ref of="Channel"() -> (w396:refnum<vi>)
        n143 = call "Switch Display.vi"("error in"=w397, "Boolean"=w396) -> ("error out"=w398:errorcluster)  [unwired: 9 in]
      }
      frame "Signal Type" {
        # "語音點選波型"
        n144 = control-ref of="Signal Type"() -> (w399:refnum<vi>)
        n145 = call "Switch Display.vi"("error in"=w401, "Boolean"=w399) -> ("error out"=w400:errorcluster)  [unwired: 9 in]
      }
      frame "Exit" {
        # "結束程式"
        n146 = Variant To Data(error in=w408, type=FALSE, Variant=w407) -> (data=w405:bool, error out=w409:errorcluster)
        n147 = case shown="True" w405 {
          tunnel: w409 -> [w411 w414]
          tunnel: [w411 w413] -> w403
          frame False {
          }
          frame True {
            n148 = control-ref of="Stop"() -> (w412:refnum<vi>)
            n149 = call "Switch Display.vi"("error in"=w414, "Boolean"=w412) -> ("error out"=w413:errorcluster)  [unwired: 9 in]
          }
        }
        n150 = call "Callback Event(FGV).vi"("Method"=enum16{"Destroy", "Put", "Get"}."Destroy", "error in"=w403) -> ("error out"=w402:errorcluster)  [unwired: 8 in, 1 out]
      }
    }
    n151 = call "Structure Error Handle.vi"("error in"=w307) -> ("error out"=w306:errorcluster)  [unwired: 10 in]
  }
  n152 = control-ref of="This VI"() -> (w1:refnum<vi>)
  n153 = Merge Errors(w4, w3) -> (w2:errorcluster)
  n154 = call "Close Front Panel.vi"("error in"=w2, "reference"=w1) -> ()  [unwired: 9 in, 1 out]
